vi "写入外设配置.vi"(8 "error in (no error)":errorcluster, 10 "外设配置":T1 {"总氮x公式0" items=["0", "1"]; "光谱仪类型" items=["1型", "2型", "3型", "2型氙灯联控"]; "泵阀量" items=["9通"=9, "10通"=10, "12通"=12]; "泵类型" items=["1型", "2型", "sy04型+旋转阀"]}, 11 "MB session in":refnum<class "MB_Master.lvclass">) -> (0 "error out":errorcluster, 3 "MB session out":refnum<class "MB_Master.lvclass">)   [LabVIEW 2016, in "斯坦道氨氮.lvlib"]
uses:
  <vilib>/Plasmionique/MB Master/MB_Master/MB_Master.lvclass
  <vilib>/Plasmionique/MB Master/MB_Master_Serial/MB_Master_Serial.lvclass
  C:/Program Files (x86)/National Instruments/LabVIEW 2016/vi.lib/Plasmionique/MB Master/MB_Master/MB_Master.lvclass
  <vilib>/Plasmionique/MB Master/MB Master.lvlib
  <vilib>/Utility/VariantDataType/VariantType.lvlib
panel:
  in  "U32":u32
  in  "SGL":sgl
  in  "U16":u16
  in  "U8":u8
  in  "VISA Resource":refnum<visa-resource-name>
  in  "引用选择":enum16{"MB引用", "自建引用"}(ring)
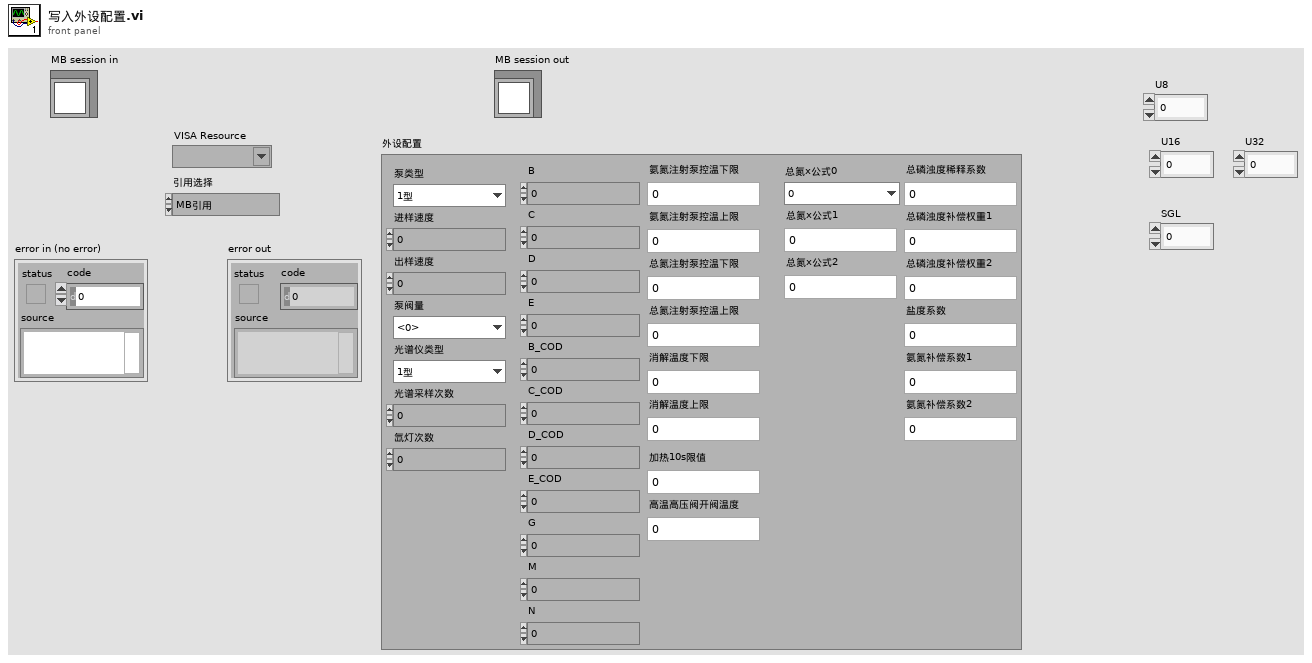
[diagram p1: front panel]
types:
  T1 = cluster{"泵类型":u8, "进样速度":u32, "出样速度":u32, "泵阀量":u8, "光谱仪类型":u8, "光谱采样次数":u8, "氙灯次数":u8, "B":u16, "C":u16, "D":u16, "E":u16, "B_COD":u16, "C_COD":u16, "D_COD":u16, "E_COD":u16, "G":u16, "M":u16, "N":u16, "氨氮注射泵控温下限":sgl, "氨氮注射泵控温上限":sgl, "总氮注射泵控温下限":sgl, "总氮注射泵控温上限":sgl, "消解温度下限":sgl, "消解温度上限":sgl, "加热10s限值":sgl, "高温高压阀开阀温度":sgl, "总氮x公式0":u8, "总氮x公式1":sgl, "总氮x公式2":sgl, "总磷浊度稀释系数":sgl, "总磷浊度补偿权重1":sgl, "总磷浊度补偿权重2":sgl, "盐度系数":sgl, "氨氮补偿系数1":sgl, "氨氮补偿系数2":sgl}
  T2 = typedef "VariantType.lvlib/Type.ctl" = enum8{"Invalid Type", "Void", "I8", "I16", "I32", "I64", "U8", "U16", "U32", "U64", "Single Float", "Double Float", "Extended Float", "Single Complex", "Double Complex", "Extended Complex", "Enum U8", "Enum U16", "Enum U32", "Enum U64", "Single Float With Unit", "Double Float With Unit", "Extended Float With Unit", "Single Complex with Unit", "Double Complex with Unit", "Extended Complex with Unit", "Boolean", "String", "Path", "Picture", "Tag", "Array", "Cluster", "Variant", "LV Variant", "Waveform", "Timestamp", "Digital Waveform", "Digital Data", "ExpressData", "Refnum", "External Data", "VI", "Poly VI", "LabVIEW Class Instance", "Fixed Point"}
  T3 = cluster{"baud rate (bps)":u32, "stop bits":u16, "parity":u16, "flow control":u16, "timeout":u32, "retries":i32}
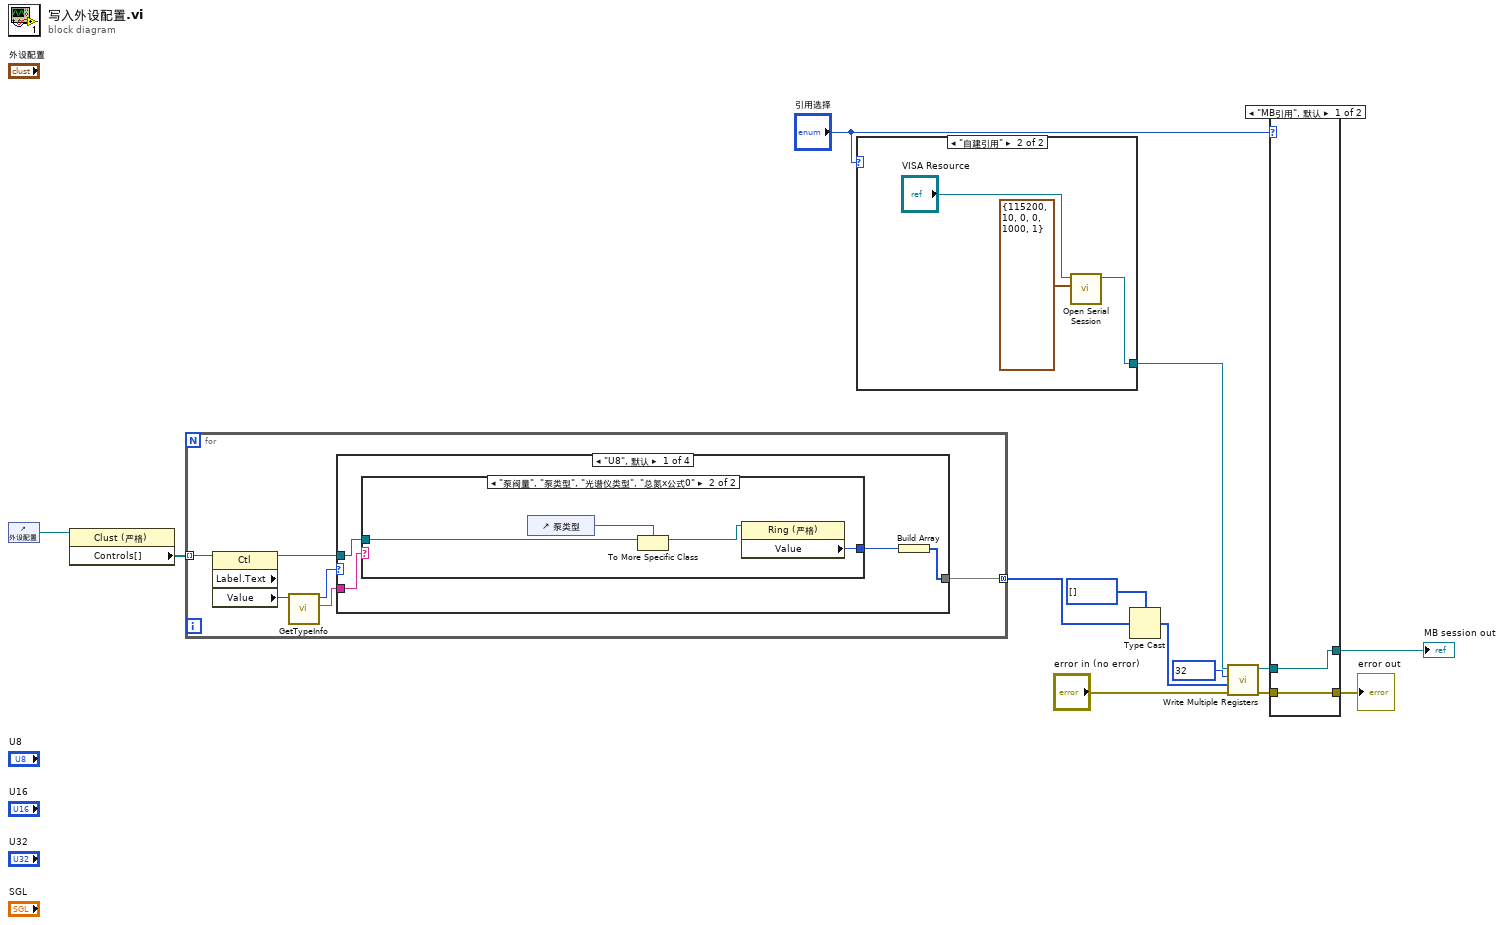
[diagram p0: block diagram]
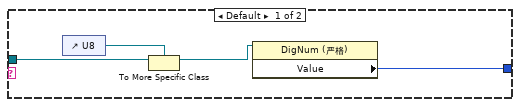
[diagram p2: hidden frame]
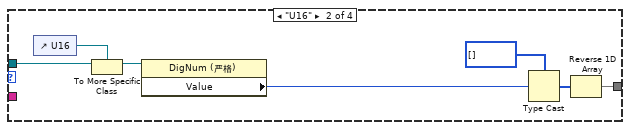
[diagram p3: hidden frame]
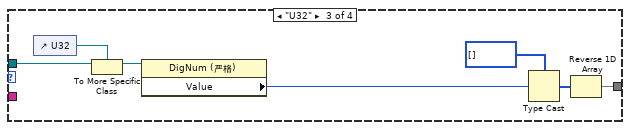
[diagram p4: hidden frame]
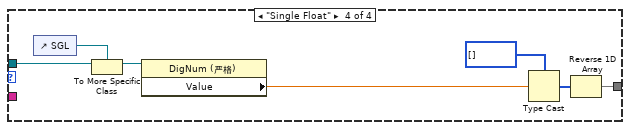
[diagram p5: hidden frame]
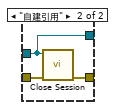
[diagram p6: hidden frame]
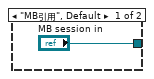
[diagram p7: hidden frame]
diagram:
  n1 = control-ref of="外设配置"() -> (w5:refnum<vi>)
  n2 = property class="Clust (严格)"(reference=w5) -> ("Controls[]"=w4:refnum<vi>[])  [unwired: 1 in, 2 out]
  n3 = for {
    tunnel: w4 -> [w19] mode=indexing
    tunnel: [w15] -> w2 mode=concatenating
    n4 = property class="Ctl" props=["Label", "Text", "Value"](reference=w19) -> (reference out=w16:refnum<vi>, "Value"=w18:variant)  [unwired: 1 in, 2 out]
    n5 = call <vilib>:"GetTypeInfo.vi"("Variant"=w18) -> ("Name"=w14:string, "Type Enum"=w17:T2)  [unwired: 6 in, 3 out]
    n6 = case shown="\"U8\", 默认" w17 {
      tunnel: w16 -> [w21 w38 w45 w52]
      tunnel: [w23 w32 w39 w46] -> w15
      tunnel: w14 -> [w22 _ _ _]
      frame "U8", Default {
        n7 = case shown="\"泵阀量\", \"泵类型\", \"光谱仪类型\", \"总氮x公式0\"" w22 {
          tunnel: w21 -> [w26 w31]
          tunnel: [w24 w28] -> w20
          frame Default {
            n8 = control-ref of="U8"() -> (w27:refnum<vi>)
            n9 = To More Specific Class(target class=w27, reference=w26) -> (specific class reference=w25:refnum<vi>)  [unwired: 1 in, 1 out]
            n10 = property class="DigNum (严格)"(reference=w25) -> ("Value"=w24:u8)  [unwired: 1 in, 2 out]
          }
          frame "泵阀量", "泵类型", "光谱仪类型", "总氮x公式0" {
            n11 = control-ref of="泵类型"() -> (w30:refnum<vi>)
            n12 = To More Specific Class(target class=w30, reference=w31) -> (specific class reference=w29:refnum<vi>)  [unwired: 1 in, 1 out]
            n13 = property class="Ring (严格)"(reference=w29) -> ("Value"=w28:u8)  [unwired: 1 in, 2 out]
          }
        }
        n14 = Build Array(w20) -> (w23:u8[])
      }
      frame "U16" {
        n15 = control-ref of="U16"() -> (w37:refnum<vi>)
        n16 = To More Specific Class(target class=w37, reference=w38) -> (specific class reference=w36:refnum<vi>)  [unwired: 1 in, 1 out]
        n17 = property class="DigNum (严格)"(reference=w36) -> ("Value"=w33:u16)  [unwired: 1 in, 2 out]
        n18 = Type Cast(type=u8[] [], x=w33) -> (*(type *) &x=w35:u8[])
        n19 = Reverse 1D Array(array=w35) -> (reversed array=w32:u8[])
      }
      frame "U32" {
        n20 = control-ref of="U32"() -> (w44:refnum<vi>)
        n21 = To More Specific Class(target class=w44, reference=w45) -> (specific class reference=w43:refnum<vi>)  [unwired: 1 in, 1 out]
        n22 = property class="DigNum (严格)"(reference=w43) -> ("Value"=w40:u32)  [unwired: 1 in, 2 out]
        n23 = Type Cast(type=u8[] [], x=w40) -> (*(type *) &x=w42:u8[])
        n24 = Reverse 1D Array(array=w42) -> (reversed array=w39:u8[])
      }
      frame "Single Float" {
        n25 = control-ref of="SGL"() -> (w51:refnum<vi>)
        n26 = To More Specific Class(target class=w51, reference=w52) -> (specific class reference=w50:refnum<vi>)  [unwired: 1 in, 1 out]
        n27 = property class="DigNum (严格)"(reference=w50) -> ("Value"=w47:sgl)  [unwired: 1 in, 2 out]
        n28 = Type Cast(type=u8[] [], x=w47) -> (*(type *) &x=w49:u8[])
        n29 = Reverse 1D Array(array=w49) -> (reversed array=w46:u8[])
      }
    }
  }
  n30 = case shown="\"自建引用\"" "引用选择" {
    tunnel: ["MB session in" w56] -> w11
    frame "MB引用", Default {
    }
    frame "自建引用" {
      n31 = call <vilib>:"Open Serial Session.vi"("Serial Config"=T3 {"baud rate (bps)"=115200, "stop bits"=10, "parity"=0, "flow control"=0, "timeout"=1000, "retries"=1}, "VISA Resource"="VISA Resource") -> ("MB_Serial session"=w56:refnum<class "MB_Master_Serial.lvclass">)  [unwired: 8 in, 1 out]
    }
  }
  n32 = Type Cast(type=u16[] [], x=w2) -> (*(type *) &x=w1:u16[])
  n33 = call <vilib>:"Write Multiple Registers.vi"("error in (no error)"="error in (no error)", "values"=w1, "starting address"=u16 32, "MB session in"=w11) -> ("error out"=w8:errorcluster, "MB session out"=w10:refnum<class "MB_Master.lvclass">)  [unwired: 6 in]
  n34 = case shown="\"MB引用\", 默认" "引用选择" {
    tunnel: w10 -> [w57 w59]
    tunnel: w8 -> [w58 w61]
    tunnel: [w58 w60] -> w7
    tunnel: [w57 w59] -> w6
    frame "MB引用", Default {
    }
    frame "自建引用" {
      n35 = call-dynamic "Close Session.vi"("error in (no error)"=w61, "MB session in"=w59) -> ("error out"=w60:errorcluster)  [unwired: 9 in]
    }
  }
  "MB session out" <- w6
  "error out" <- w7
